vi "6.0.0_Finalization_good_unit.vi"(7 "Data in":T1, 8 "error in (no error)":errorcluster, 9 "AllControls In":T2, 10 "?":T3, 11 "Message Queue out":T4) -> (0 "error out":errorcluster, 1 "Flow":string, 2 "Data":T3, 3 "Message Queue Out":T4, 5 "Data out":T1)   [LabVIEW 2017]
uses:
  Depends/AMC/subVIs/TypeDefs/amc_Message Queue.ctl
  Depends/AMC/subVIs/TypeDefs/amc_Message.ctl
  Depends/Tools/Keyed Array/Tools_KeyedArray KeyedArray.ctl
  Ctrls/Data.ctl
  Ctrls/AllControls.ctl
  Ctrls/CSV_Data.ctl
  DIPC 692 Daemon API/typdef/device_mode.ctl
  Ctrls/PathChoose.ctl
  DIPC 692 Daemon API/typdef/read_nvm_section.ctl
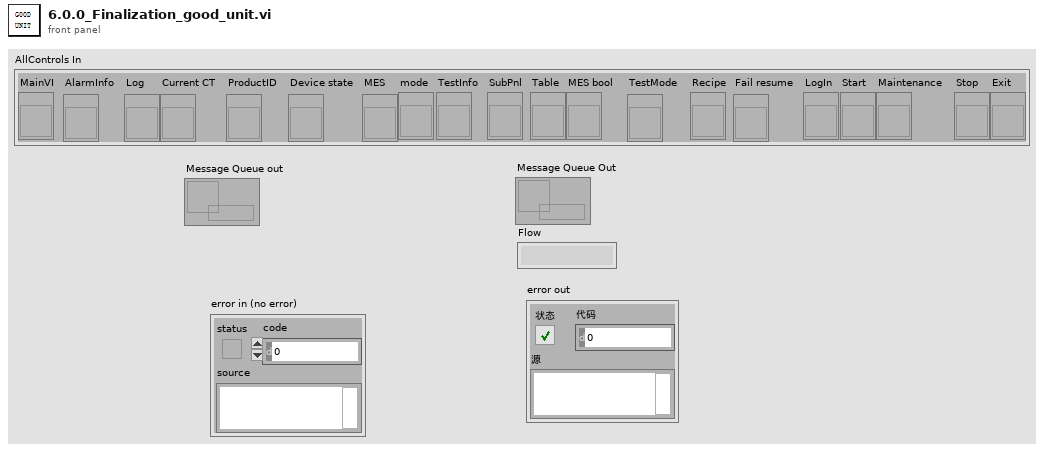
[diagram p1: front panel]
types:
  T1 = typedef "CSV_Data.ctl" = cluster{"Initialisation":cluster{"LMT - Connect UUT (con COM)":string, "LMT - Software Version (rrel)":string, "LMT - Write SKU file (wskuc)":string, "LMT - SKU file name":string, "Connect UUT DDM":string, "Read DDM EOL Timestamp - Mode":string, "Read DDM EOL Timestamp - Timestamp":string, "Read DDM EOL Timestamp - Rig ID":string, "Read DDM EOL Timestamp - Passmark ID":string, "Read DDM EOL Timestamp - Passmark Rev":string, "Software Version before flashing":string, "Read Hardware Serial":string, "UUT DDM SN":string, "Compare DDM SN with MES SN":string, "Backup PCBA Calibration EEPROM Response - CAL":string, "Flash Firmware Version":string, "Check SW Version":string, "Read DDM SW Version after flashing":string, "Set SKU Config":string, "Ready Status":string, "Set Device Mode to EOL":string, "DDM Parameter - Voltage":string, "DDM Parameter - Current":string, "DDM Parameter - Power":string, "DDM Parameter - Speed":string, "DDM Parameter - Pressure":string, "Tester Parameter - Voltage":string, "Tester Parameter - Current":string, "Tester Parameter - Power":string, "Tester Parameter - Ambient Pressure":string, "Tester Parameter - Ambient Temperature":string, "Calculated Parameter - DDM Pressure Corrected":string, "Calculated Parameter - DDM Real Power":string, "Calculated Parameter - Delta V":string}, "BEMF_Calibration":cluster{"Calibration Result - eol_cold_bemf_temp":string, "DDM Ambient Temp":string, "Restriction Plate Diameter":string, "Calibration Result - eol_bemf_mp_cold_coef_a":string, "Calibration Result - eol_bemf_mp_cold_coef_b":string, "Calibration Result - eol_bemf_mp_cold_coef_c":string, "Calibration Result - eol_bemf_lsi_cold_ref_coeffs":string, "Get - Calibration Result - eol_bemf_lsi_speed":string, "Get - Calibration Result - eol_bemf_lsi_integral_0":string, "Calibration Result - eol_bemf_lsi_integral_1":string, "Get - Calibration Result - eol_bemf_lsi_integral_2":string, "Get - Calibration Result - eol_cold_bemf":string, "Get - Calibration Result - eol_cold_bemf_fisf":string, "Finalise Calibration":string, "Compare -Calibration Result - eol_cold_bemf":string, "Compare -Calibration Result - eol_cold_bemf_fisf":string}, "ECO":cluster{"Reset Power Tune":string, "Reset BEMF FISF Calibration":string, "Restriction Plate Diameter":string, "ECO - Stabilisation Time":string, "ECO - DDM Parameter - Voltage":string, "ECO - DDM Parameter - Current":string, "ECO - DDM Parameter - Power":string, "ECO - DDM Parameter - Measured Power":string, "ECO - DDM Parameter - Speed":string, "ECO - DDM Parameter - Pressure":string, "ECO - Tester Parameter - Voltage":string, "ECO - Tester Parameter - Current":string, "ECO - Tester Parameter - Power":string, "ECO - Tester Parameter - Ambient Pressure":string, "ECO - Tester Parameter - Ambient Temperature":string, "ECO - Tester Parameter - Ambient Humidity":string, "ECO - Calculated Parameter - DDM Pressure Corrected":string, "ECO - Calculated Parameter - DDM Real Power":string, "ECO - Calculated Parameter - Delta V":string, "ECO - Calculated Parameter - Flowrate":string, "ECO - Calculated Parameter - Airwatt":string, "ECO - Formula":string, "PT ECO - Power Tune Mode Status":string}, "BOOST":cluster{"Restriction Plate Diameter":string, "BOOST - Stabilisation Time":string, "BOOST - DDM Parameter - Voltage":string, "BOOST - DDM Parameter - Current":string, "BOOST - DDM Parameter - Power":string, "BOOST - DDM Parameter - Measured Power":string, "BOOST - DDM Parameter - Speed":string, "BOOST - DDM Parameter - Pressure":string, "BOOST - Tester Parameter - Voltage":string, "BOOST - Tester Parameter - Current":string, "BOOST - Tester Parameter - Power":string, "BOOST - Tester Parameter - Ambient Pressure":string, "BOOST - Tester Parameter - Ambient Temperature":string, "BOOST - Tester Parameter - Ambient Humidity":string, "BOOST - Calculated Parameter - DDM Pressure Corrected":string, "BOOST - Calculated Parameter - DDM Real Power":string, "BOOST - Calculated Parameter - Delta V":string, "BOOST - Calculated Parameter - Flowrate":string, "BOOST - Calculated Parameter - Airwatt":string, "BOOST - Get AM Presence":string, "Air Muscle Turn Off Status":string, "BOOST - Air Muscle Calculated Parameter - Airwatt B":string, "BOOST - Air Muscle Calculate Airwatt Delta":string, "PT BOOST - Power Tune Mode Status":string, "Finalise Calibration":string, "ECO - Get AW Calibration value":string, "BOOST - Get AW Calibration value":string}, "MAX":cluster{"Restriction Plate Diameter":string, "MAX - Stabilisation Time":string, "Get Average Delta Tmag (LSIdelta_FISFdelta_LSItmag_FISFtmag_IIRtmag)":string, "Get Average Delta Tmag FISF":string, "MAX - DDM Parameter - Voltage":string, "MAX - DDM Parameter - Current":string, "MAX - DDM Parameter - Power":string, "MAX - DDM Parameter - Measured Power":string, "MAX - DDM Parameter - Speed":string, "MAX - DDM Parameter - Pressure":string, "MAX - Tester Parameter - Voltage":string, "MAX - Tester Parameter - Current":string, "MAX - Tester Parameter - Power":string, "MAX - Tester Parameter - Ambient Pressure":string, "MAX - Tester Parameter - Ambient Temperature":string, "MAX - Tester Parameter - Ambient Humidity":string, "MAX - Calculated Parameter - DDM Pressure Corrected":string, "MAX - Calculated Parameter - DDM Real Power":string, "MAX - Calculated Parameter - Delta V":string, "MAX - Calculated Parameter - Flowrate":string, "MAX - Calculated Parameter - Airwatt":string, "MAX_FISF_Check_Average_Delta_Tmag":string, "MAX - FISF - BEMF Finetune Result":string, "MAX tune - Delta P1":string, "MAX tune - Calculated Parameter - Airwatt":string, "Calculate Delta Airwatts - MAX finetune - Delta P2":string, "MAX finetune - DDM Parameter - Voltage":string, "MAX finetune - DDM Parameter - Current":string, "MAX finetune - DDM Parameter - Power":string, "MAX finetune - DDM Parameter - Measured Power":string, "MAX finetune - DDM Parameter - Speed":string, "MAX finetune - DDM Parameter - Pressure":string, "MAX finetune - Tester Parameter - Voltage":string, "MAX finetune - Tester Parameter - Current":string, "MAX finetune - Tester Parameter - Power":string, "MAX finetune - Tester Parameter - Ambient Pressure":string, "MAX finetune - Tester Parameter - Ambient Temperature":string, "MAX finetune - Tester Parameter - Ambient Humidity":string, "MAX finetune - Calculated Parameter - DDM Pressure Corrected":string, "MAX finetune - Calculated Parameter - DDM Real Power":string, "MAX finetune - Calculated Parameter - Delta V":string, "MAX finetune - Calculated Parameter - Flowrate":string, "MAX finetune - Calculated Parameter - Airwatt":string, "Check Derate Result":string, "Delta Tmag FISF":string, "Get Hot BEMF Result":string, "Calculate delta Pressure":string, "Finalise Calibration":string, "Calculate & Check Delta BEMF":string, "Delta P Airwatts Value":string}, "LL":cluster{"DDM Ambient Temp":string, "Restriction Plate Diameter":string, "LL - DDM Parameter - Voltage":string, "LL - DDM Parameter - Current":string, "LL - DDM Parameter - Power":string, "LL - DDM Parameter - Measured Power":string, "LL - DDM Parameter - Speed":string, "LL - DDM Parameter - Pressure":string, "LL - Tester Parameter - Voltage":string, "LL - Tester Parameter - Current":string, "LL - Tester Parameter - Power":string, "LL - DDM Real Power":string, "LL - Calibrate Task Detect LL":string}, "HL":cluster{"HL - DDM Parameter - Voltage":string, "HL - DDM Parameter - Current":string, "HL - DDM Parameter - Power":string, "HL - DDM Parameter - Measured Power":string, "HL - DDM Parameter - Speed":string, "HL - DDM Parameter - Pressure":string, "HL - Tester Parameter - Voltage":string, "HL - Tester Parameter - Current":string, "HL - Tester Parameter - Power":string, "HL - DDM Real Power":string, "HL - Calibrate Task Detect HL":string}, "LH":cluster{"Restriction Plate Diameter":string, "LH - DDM Parameter - Voltage":string, "LH - DDM Parameter - Current":string, "LH - DDM Parameter - Power":string, "LH - DDM Parameter - Measured Power":string, "LH - DDM Parameter - Speed":string, "LH - DDM Parameter - Pressure":string, "LH - Tester Parameter - Voltage":string, "LH - Tester Parameter - Current":string, "LH - Tester Parameter - Power":string, "LH - DDM Real Power":string, "LH - Calibrate Task Detect LH":string}, "HH":cluster{"HH - DDM Parameter - Voltage":string, "HH - DDM Parameter - Current":string, "HH - DDM Parameter - Power":string, "HH - DDM Parameter - Measured Power":string, "HH - DDM Parameter - Speed":string, "HH - DDM Parameter - Pressure":string, "HH - Tester Parameter - Voltage":string, "HH - Tester Parameter - Current":string, "HH - Tester Parameter - Power":string, "HH - DDM Real Power":string, "HH - Calibrate Task Detect HH":string}, "Inlet Blockage Calibration":cluster{"Inlet Blockage Calibration - DDM Parameter - Voltage":string, "Inlet Blockage Calibration - DDM Parameter - Current":string, "Inlet Blockage Calibration - DDM Parameter - Power":string, "Inlet Blockage Calibration - DDM Parameter - Measured Power":string, "Inlet Blockage Calibration - DDM Parameter - Speed":string, "Inlet Blockage Calibration - DDM Parameter - Pressure":string, "Inlet Blockage Calibration - Tester Parameter - Voltage":string, "Inlet Blockage Calibration - Tester Parameter - Current":string, "Inlet Blockage Calibration - Tester Parameter - Power":string, "Inlet Blockage Calibration - DDM Real Power":string, "Calibration Inlet Blockage_E":string, "Finalise Calibration":string, "Get Task Detect LL":string, "Get Task Detect HL":string, "Get Task Detect LH":string, "Get Task Detect HH":string, "Calibration Inlet Blockage":string, "Calibration eol cold bemf temp":string}, "GOOD":cluster{"GOOD UNIT - Clear EEPROM Error Log":string, "GOOD UNIT - Write Product Timestamp - Mode":string, "GOOD UNIT - Write Product Timestamp - Timestamp":string, "GOOD UNIT - Write Product Timestamp - Rig ID":string, "GOOD UNIT - Write Product Timestamp - Passmark ID":string, "GOOD UNIT - Write Product Timestamp - Passmark Rev":string, "GOOD UNIT - Set Device Mode to PROD":string, "GOOD UNIT - Backup PCBA Calibration EEPROM Response":string, "GOOD UNIT - Check Security Bit":string, "GOOD UNIT - Set Calibration Lock":string, "GOOD UNIT - Get_Calibration_Lock":string, "GOOD UNIT - Disconnect UUT":string}, "NG":cluster{"NG UNIT - Read NVM Error":string, "NG UNIT - Set Device Mode to FCT":string, "NG UNIT - Backup PCBA Calibration EEPROM Response - CAL":string, "NG UNIT - Backup PCBA Calibration EEPROM Response - ERROR":string, "NG UNIT - Backup PCBA Calibration EEPROM Response - USAGE":string, "NG UNIT - Disconnect UUT":string}, "SN":string, "Table":string[][], "Count":cluster{"Total":i32, "OK":i32, "NG":i32, "Yield":dbl}, "Start Time":timestamp, "daemon reference":refnum<k5>, "CT":dbl, "Config":string[][], "OK/NG":bool, "Station ID":string, "MES DDM SN":string, "MES PCBA SN":string, "Retest":string, "UID":string, "Initialisation_Status":cluster{"LMT - Connect UUT (con COM)":string, "LMT - Software Version (rrel)":string, "LMT - Write SKU file (wskuc)":string, "LMT - SKU file name":string, "Connect UUT DDM":string, "Read DDM EOL Timestamp - Mode":string, "Read DDM EOL Timestamp - Timestamp":string, "Read DDM EOL Timestamp - Rig ID":string, "Read DDM EOL Timestamp - Passmark ID":string, "Read DDM EOL Timestamp - Passmark Rev":string, "Software Version before flashing":string, "Read Hardware Serial":string, "UUT DDM SN":string, "Compare DDM SN with MES SN":string, "Backup PCBA Calibration EEPROM Response - CAL":string, "Flash Firmware Version":string, "Check SW Version":string, "Read DDM SW Version after flashing":string, "Set SKU Config":string, "Ready Status":string, "Set Device Mode to EOL":string, "DDM Parameter - Voltage":string, "DDM Parameter - Current":string, "DDM Parameter - Power":string, "DDM Parameter - Speed":string, "DDM Parameter - Pressure":string, "Tester Parameter - Voltage":string, "Tester Parameter - Current":string, "Tester Parameter - Power":string, "Tester Parameter - Ambient Pressure":string, "Tester Parameter - Ambient Temperature":string, "Calculated Parameter - DDM Pressure Corrected":string, "Calculated Parameter - DDM Real Power":string, "Calculated Parameter - Delta V":string}, "BEMF_Calibration_Status":cluster{"Calibration Result - eol_cold_bemf_temp":string, "DDM Ambient Temp":string, "Restriction Plate Diameter":string, "Calibration Result - eol_bemf_mp_cold_coef_a":string, "Calibration Result - eol_bemf_mp_cold_coef_b":string, "Calibration Result - eol_bemf_mp_cold_coef_c":string, "Calibration Result - eol_bemf_lsi_cold_ref_coeffs":string, "Get - Calibration Result - eol_bemf_lsi_speed":string, "Get - Calibration Result - eol_bemf_lsi_integral_0":string, "Calibration Result - eol_bemf_lsi_integral_1":string, "Get - Calibration Result - eol_bemf_lsi_integral_2":string, "Get - Calibration Result - eol_cold_bemf":string, "Get - Calibration Result - eol_cold_bemf_fisf":string, "Finalise Calibration":string, "Compare -Calibration Result - eol_cold_bemf":string, "Compare -Calibration Result - eol_cold_bemf_fisf":string}, "ECO_Status":cluster{"Reset Power Tune":string, "Reset BEMF FISF Calibration":string, "Restriction Plate Diameter":string, "ECO - Stabilisation Time":string, "ECO - DDM Parameter - Voltage":string, "ECO - DDM Parameter - Current":string, "ECO - DDM Parameter - Power":string, "ECO - DDM Parameter - Measured Power":string, "ECO - DDM Parameter - Speed":string, "ECO - DDM Parameter - Pressure":string, "ECO - Tester Parameter - Voltage":string, "ECO - Tester Parameter - Current":string, "ECO - Tester Parameter - Power":string, "ECO - Tester Parameter - Ambient Pressure":string, "ECO - Tester Parameter - Ambient Temperature":string, "ECO - Tester Parameter - Ambient Humidity":string, "ECO - Calculated Parameter - DDM Pressure Corrected":string, "ECO - Calculated Parameter - DDM Real Power":string, "ECO - Calculated Parameter - Delta V":string, "ECO - Calculated Parameter - Flowrate":string, "ECO - Calculated Parameter - Airwatt":string, "ECO - Formula":string, "PT ECO - Power Tune Mode Status":string}, "BOOST_Status":cluster{"Restriction Plate Diameter":string, "BOOST - Stabilisation Time":string, "BOOST - DDM Parameter - Voltage":string, "BOOST - DDM Parameter - Current":string, "BOOST - DDM Parameter - Power":string, "BOOST - DDM Parameter - Measured Power":string, "BOOST - DDM Parameter - Speed":string, "BOOST - DDM Parameter - Pressure":string, "BOOST - Tester Parameter - Voltage":string, "BOOST - Tester Parameter - Current":string, "BOOST - Tester Parameter - Power":string, "BOOST - Tester Parameter - Ambient Pressure":string, "BOOST - Tester Parameter - Ambient Temperature":string, "BOOST - Tester Parameter - Ambient Humidity":string, "BOOST - Calculated Parameter - DDM Pressure Corrected":string, "BOOST - Calculated Parameter - DDM Real Power":string, "BOOST - Calculated Parameter - Delta V":string, "BOOST - Calculated Parameter - Flowrate":string, "BOOST - Calculated Parameter - Airwatt":string, "BOOST - Get AM Presence":string, "Air Muscle Turn Off Status":string, "BOOST - Air Muscle Calculated Parameter - Airwatt B":string, "BOOST - Air Muscle Calculate Airwatt Delta":string, "PT BOOST - Power Tune Mode Status":string, "Finalise Calibration":string, "ECO - Get AW Calibration value":string, "BOOST - Get AW Calibration value":string}, "MAX_Status":cluster{"Restriction Plate Diameter":string, "MAX - Stabilisation Time":string, "Get Average Delta Tmag (LSIdelta_FISFdelta_LSItmag_FISFtmag_IIRtmag)":string, "Get Average Delta Tmag FISF":string, "MAX - DDM Parameter - Voltage":string, "MAX - DDM Parameter - Current":string, "MAX - DDM Parameter - Power":string, "MAX - DDM Parameter - Measured Power":string, "MAX - DDM Parameter - Speed":string, "MAX - DDM Parameter - Pressure":string, "MAX - Tester Parameter - Voltage":string, "MAX - Tester Parameter - Current":string, "MAX - Tester Parameter - Power":string, "MAX - Tester Parameter - Ambient Pressure":string, "MAX - Tester Parameter - Ambient Temperature":string, "MAX - Tester Parameter - Ambient Humidity":string, "MAX - Calculated Parameter - DDM Pressure Corrected":string, "MAX - Calculated Parameter - DDM Real Power":string, "MAX - Calculated Parameter - Delta V":string, "MAX - Calculated Parameter - Flowrate":string, "MAX - Calculated Parameter - Airwatt":string, "MAX_FISF_Check_Average_Delta_Tmag":string, "MAX - FISF - BEMF Finetune Result":string, "MAX tune - Delta P1":string, "MAX tune - Calculated Parameter - Airwatt":string, "Calculate Delta Airwatts - MAX finetune - Delta P2":string, "MAX finetune - DDM Parameter - Voltage":string, "MAX finetune - DDM Parameter - Current":string, "MAX finetune - DDM Parameter - Power":string, "MAX finetune - DDM Parameter - Measured Power":string, "MAX finetune - DDM Parameter - Speed":string, "MAX finetune - DDM Parameter - Pressure":string, "MAX finetune - Tester Parameter - Voltage":string, "MAX finetune - Tester Parameter - Current":string, "MAX finetune - Tester Parameter - Power":string, "MAX finetune - Tester Parameter - Ambient Pressure":string, "MAX finetune - Tester Parameter - Ambient Temperature":string, "MAX finetune - Tester Parameter - Ambient Humidity":string, "MAX finetune - Calculated Parameter - DDM Pressure Corrected":string, "MAX finetune - Calculated Parameter - DDM Real Power":string, "MAX finetune - Calculated Parameter - Delta V":string, "MAX finetune - Calculated Parameter - Flowrate":string, "MAX finetune - Calculated Parameter - Airwatt":string, "Check Derate Result":string, "Delta Tmag FISF":string, "Get Hot BEMF Result":string, "Calculate delta Pressure":string, "Finalise Calibration":string, "Calculate & Check Delta BEMF":string, "Delta P Airwatts Value":string}, "LL_Status":cluster{"DDM Ambient Temp":string, "Restriction Plate Diameter":string, "LL - DDM Parameter - Voltage":string, "LL - DDM Parameter - Current":string, "LL - DDM Parameter - Power":string, "LL - DDM Parameter - Measured Power":string, "LL - DDM Parameter - Speed":string, "LL - DDM Parameter - Pressure":string, "LL - Tester Parameter - Voltage":string, "LL - Tester Parameter - Current":string, "LL - Tester Parameter - Power":string, "LL - DDM Real Power":string, "LL - Calibrate Task Detect LL":string}, "HL_Status":cluster{"HL - DDM Parameter - Voltage":string, "HL - DDM Parameter - Current":string, "HL - DDM Parameter - Power":string, "HL - DDM Parameter - Measured Power":string, "HL - DDM Parameter - Speed":string, "HL - DDM Parameter - Pressure":string, "HL - Tester Parameter - Voltage":string, "HL - Tester Parameter - Current":string, "HL - Tester Parameter - Power":string, "HL - DDM Real Power":string, "HL - Calibrate Task Detect HL":string}, "LH_Status":cluster{"Restriction Plate Diameter":string, "LH - DDM Parameter - Voltage":string, "LH - DDM Parameter - Current":string, "LH - DDM Parameter - Power":string, "LH - DDM Parameter - Measured Power":string, "LH - DDM Parameter - Speed":string, "LH - DDM Parameter - Pressure":string, "LH - Tester Parameter - Voltage":string, "LH - Tester Parameter - Current":string, "LH - Tester Parameter - Power":string, "LH - DDM Real Power":string, "LH - Calibrate Task Detect LH":string}, "HH_Status":cluster{"HH - DDM Parameter - Voltage":string, "HH - DDM Parameter - Current":string, "HH - DDM Parameter - Power":string, "HH - DDM Parameter - Measured Power":string, "HH - DDM Parameter - Speed":string, "HH - DDM Parameter - Pressure":string, "HH - Tester Parameter - Voltage":string, "HH - Tester Parameter - Current":string, "HH - Tester Parameter - Power":string, "HH - DDM Real Power":string, "HH - Calibrate Task Detect HH":string}, "Inlet Blockage Calibration_Status":cluster{"Inlet Blockage Calibration - DDM Parameter - Voltage":string, "Inlet Blockage Calibration - DDM Parameter - Current":string, "Inlet Blockage Calibration - DDM Parameter - Power":string, "Inlet Blockage Calibration - DDM Parameter - Measured Power":string, "Inlet Blockage Calibration - DDM Parameter - Speed":string, "Inlet Blockage Calibration - DDM Parameter - Pressure":string, "Inlet Blockage Calibration - Tester Parameter - Voltage":string, "Inlet Blockage Calibration - Tester Parameter - Current":string, "Inlet Blockage Calibration - Tester Parameter - Power":string, "Inlet Blockage Calibration - DDM Real Power":string, "Calibration Inlet Blockage_E":string, "Finalise Calibration":string, "Get Task Detect LL":string, "Get Task Detect HL":string, "Get Task Detect LH":string, "Get Task Detect HH":string, "Calibration Inlet Blockage":string, "Calibration eol cold bemf temp":string}, "GOOD_Status":cluster{"GOOD UNIT - Clear EEPROM Error Log":string, "GOOD UNIT - Write Product Timestamp - Mode":string, "GOOD UNIT - Write Product Timestamp - Timestamp":string, "GOOD UNIT - Write Product Timestamp - Rig ID":string, "GOOD UNIT - Write Product Timestamp - Passmark ID":string, "GOOD UNIT - Write Product Timestamp - Passmark Rev":string, "GOOD UNIT - Set Device Mode to PROD":string, "GOOD UNIT - Backup PCBA Calibration EEPROM Response":string, "GOOD UNIT - Check Security Bit":string, "GOOD UNIT - Set Calibration Lock":string, "GOOD UNIT - Get_Calibration_Lock":string, "GOOD UNIT - Disconnect UUT":string}, "NG_Status":cluster{"NG UNIT - Read NVM Error":string, "NG UNIT - Set Device Mode to FCT":string, "NG UNIT - Backup PCBA Calibration EEPROM Response - CAL":string, "NG UNIT - Backup PCBA Calibration EEPROM Response - ERROR":string, "NG UNIT - Backup PCBA Calibration EEPROM Response - USAGE":string, "NG UNIT - Disconnect UUT":string}, "SKU":string, "Plate_Diameter":string, "Alarm":string}
  T2 = typedef "AllControls.ctl" = cluster{"MainVI":refnum<vi>, "AlarmInfo":refnum<vi>, "Log":refnum<vi>, "Current CT":refnum<vi>, "ProductID":refnum<vi>, "Device state":refnum<vi>, "MES":refnum<vi>, "mode":refnum<vi>, "TestInfo":refnum<vi>, "SubPnl":refnum<vi>, "Table":refnum<vi>, "MES bool":refnum<vi>, "TestMode":refnum<vi>, "Recipe":refnum<vi>, "Fail resume":refnum<vi>, "LogIn":refnum<vi>, "Start":refnum<vi>, "Maintenance":refnum<vi>, "Stop":refnum<vi>, "Exit":refnum<vi>}
  T3 = typedef "Data.ctl" = cluster{"Initialisation":cluster{"DDM_Parameter":dbl[], "DDM_Parameter_status":bool[], "Get_Tester_Parameter":dbl[], "Get_Tester_Parameter_status":bool[], "Cal_Tester_Parameter":dbl[], "Cal_Tester_Parameter_status":bool[], "sw_version_before_status":bool, "sw_version_after_status":bool, "Set_SKU_Config_With_LMT_status":bool, "FCT_timestamp_status":bool, "LMT_Connect_to_UUT_status":bool}, "BEMF_Calibration":cluster{"Read_ambient_temperature":dbl, "Calibration_Vaule":dbl[], "Calibration_Vaule _B":dbl[], "Calibration_Vaule_status":bool[], "Calibration_Vaule_B_status":bool[]}, "ECO":cluster{"DDM_Parameter":dbl[], "DDM_Parameter_status":bool[], "Get_Tester_Parameter":dbl[], "Get_Tester_Parameter_status":bool[], "Cal_Tester_Parameter":dbl[], "Cal_Tester_Parameter_status":bool[], "DDM_Parameter_after_power_tune":dbl[], "Get_Tester_Parameter_after_power_tune":dbl[], "Cal_Tester_Parameter_after_power_tune":dbl[], "Cal_Tester_Parameter_after_power_tune_status":bool[], "Delta_P":dbl}, "BOOST":cluster{"DDM_Parameter":dbl[], "DDM_Parameter_status":bool[], "Get_Tester_Parameter":dbl[], "Get_Tester_Parameter_status":bool[], "Cal_Tester_Parameter":dbl[], "Cal_Tester_Parameter_status":bool[], "DDM_Parameter_after_power_tune":dbl[], "Get_Tester_Parameter_after_power_tune":dbl[], "Cal_Tester_Parameter_after_power_tune":dbl[], "Cal_Tester_Parameter_after_power_tune_status":bool[], "airwatts_am_off":dbl, "AW_Delta_(AM_on_and_off)":dbl, "AW_Delta_(AM_on_and_off)_Status":bool, "Delta_P":dbl}, "MAX":cluster{"Average_Tmag_Data":cluster{"LSI Delta in degC":dbl, "FISF Delta in degc":dbl, "LSI Tmag in degC":dbl, "Fisf Tmag in degC":dbl, "IIR Tmag in degC":dbl}, "DDM_Parameter":dbl[], "DDM_Parameter_status":bool[], "Get_Tester_Parameter":dbl[], "Get_Tester_Parameter_status":bool[], "Cal_Tester_Parameter":dbl[], "BEMF_Finetune":cluster{"eol_bemf_mp_cold_coef_c":dbl, "eol_cold_bemf_fisf_offset":dbl}, "AW_Tune":cluster{"delta_P1":dbl, "delta_P_Setting":dbl}, "DDM_Parameter_after_Airwatts_Tune":dbl[], "Get_Tester_Parameter_after_Airwatts_Tune":dbl[], "Cal_Tester_Parameter_after_Airwatts_Tune":dbl[], "DDM_Parameter_after_Airwatts_Finetune":dbl[], "Get_Tester_Parameter_after_Airwatts_Finetune":dbl[], "Cal_Tester_Parameter_after_Airwatts_Finetune":dbl[], "AW_Finetune":cluster{"delta_P2":dbl, "delta_P_Setting":dbl}, "Delta_Tmag_after_tune":cluster{"LSI Delta in degC":dbl, "FISF Delta in degc":dbl, "LSI Tmag in degC":dbl, "Fisf Tmag in degC":dbl, "IIR Tmag in degC":dbl}, "Hot Bemf in mV":dbl, "DDM_Pressure":dbl, "Delta_Pressure":dbl, " Cold Bemf in mV":dbl, " delta Bemf":dbl, " delta p":dbl, "Delta_Pressure_status":bool, " delta Bemf_status":bool, "LSI Delta in degC_status":bool, "FISF Delta in degc_status":bool, "Max_check_derate_status_status":bool, "Average_All_data":dbl[][], "Average_Tmag_Data_status":bool[], "Average_Tmag_Data_after_tune_status":bool[], "Cal_Tester_Parameter_status":bool[], "Cal_Tester_Parameter_status_after_Airwatts_Tune":bool[], "Cal_Tester_Parameter_status_after_Airwatts_FineTune":bool[]}, "Task_Detect_Calib":cluster{"LL":cluster{"DDM_Parameter":dbl[], "DDM_Parameter_status":bool[], "Get_Tester_Parameter":dbl[], "Get_Tester_Parameter_status":bool[], "Set_task_detect_A":dbl, "Set_task_detect_A_Status":bool}, "HL":cluster{"DDM_Parameter":dbl[], "DDM_Parameter_status":bool[], "Get_Tester_Parameter":dbl[], "Get_Tester_Parameter_status":bool[], "Set_task_detect_B":dbl, "Set_task_detect_B_Status":bool}, "LH":cluster{"DDM_Parameter":dbl[], "DDM_Parameter_status":bool[], "Get_Tester_Parameter":dbl[], "Get_Tester_Parameter_status":bool[], "Set_task_detect_C":dbl, "Set_task_detect_C_Status":bool}, "HH":cluster{"DDM_Parameter":dbl[], "DDM_Parameter_status":bool[], "Get_Tester_Parameter":dbl[], "Get_Tester_Parameter_status":bool[], "Set_task_detect_D":dbl, "Read_and_check_calibration_Status":bool[], "Set_task_detect_D_Status":bool}, "Get_eol_inlet_blockage_E":dbl, "Calib_vaule":cluster{"Get_task_detect_LL":dbl, "Get_task_detect_HL":dbl, "Get_task_detect_LH":dbl, "Get_task_detect_HH":dbl, "eol_inlet_blockage":dbl, "eol_code_bemf_temp":dbl}, "calibrated temp":dbl, "Inlet_Blockage_Calibration":cluster{"DDM_Parameter":dbl[], "DDM_Parameter_status":bool[], "Get_Tester_Parameter":dbl[], "Get_Tester_Parameter_status":bool[]}, "Get_eol_inlet_blockage_E_Status":bool}, "good":cluster{"Write_Product_TS":cluster{"TIMESTAMP":i64, "RIG_ID":i64, "PASSMARK_ID":i64, "PASSMARK_REV":i64}, "Read_Product_TS":cluster{"TIMESTAMP":i64, "RIG_ID":i64, "PASSMARK_ID":i64, "PASSMARK_REV":i64}, "Good_Check_Secuity_Bit_Stauts":bool}}
  T4 = typedef "amc_Message Queue.ctl" = refnum<queue>
  T5 = typedef "TesterInfo.ctl" = cluster{"Station Name":string, "Station Code":string, "ES NO.":string, "Tester ID":string, "PassMark Revision":string, "Rig ID":string, "Deamon_vision":string, "Project Name":string, "FFTesterPath":path, "Enable_User":bool, "Mode":enum16{"682"}, "MES":bool}
  T6 = typedef "HD Config.ctl" = cluster{" PC":cluster{"PC Address":u8[], "PC Port":i32}, "FCO":cluster{"COM":refnum<visa-resource-name>, "Baudrate":u32}, "DC Power ":cluster{"COM":refnum<visa-resource-name>, "Baudrate":u32}, "PW3336":cluster{"COM":refnum<visa-resource-name>, "Baudrate":u32}, "Lefoo":cluster{"COM":refnum<visa-resource-name>, "Baudrate":u32}, "AI Model":cluster{"COM":refnum<visa-resource-name>, "Baudrate":u32}, "DIPC":cluster{"COM":refnum<visa-resource-name>}, "RFID":cluster{"IP Address":string, "Port":u16, "Retry":u16}, "Motor":cluster{"COM":refnum<visa-resource-name>, "Baudrate":u32}, "Fail_resume_mode":bool, "GRR":bool}
  T7 = cluster{"TIMESTAMP":string, "RIG_ID":string, "PASSMARK_ID":string, "PASSMARK_REV":string}
  T8 = cluster{"TIMESTAMP":i64, "RIG_ID":i64, "PASSMARK_ID":i64, "PASSMARK_REV":i64}
  T9 = typedef "device_mode.ctl" = enum16{"FCT", "EOL", "PROD"}
  T10 = typedef "PathChoose.ctl" = enum16{"OperatorLog", "AutoRunLog", "AlmLog", "TestData", "AllTestData", "backup_nvm", "backup_before_flashing"}
  T11 = enum16{"open", "replace", "create", "open or create", "replace or create", "replace or create with confirmation"}
  T12 = typedef "read_nvm_section.ctl" = enum16{"CAL", "ERROR", "USAGE"}
  T13 = cluster{"[0]":i64, "[1]":i64, "[2]":i64, "[3]":i64}
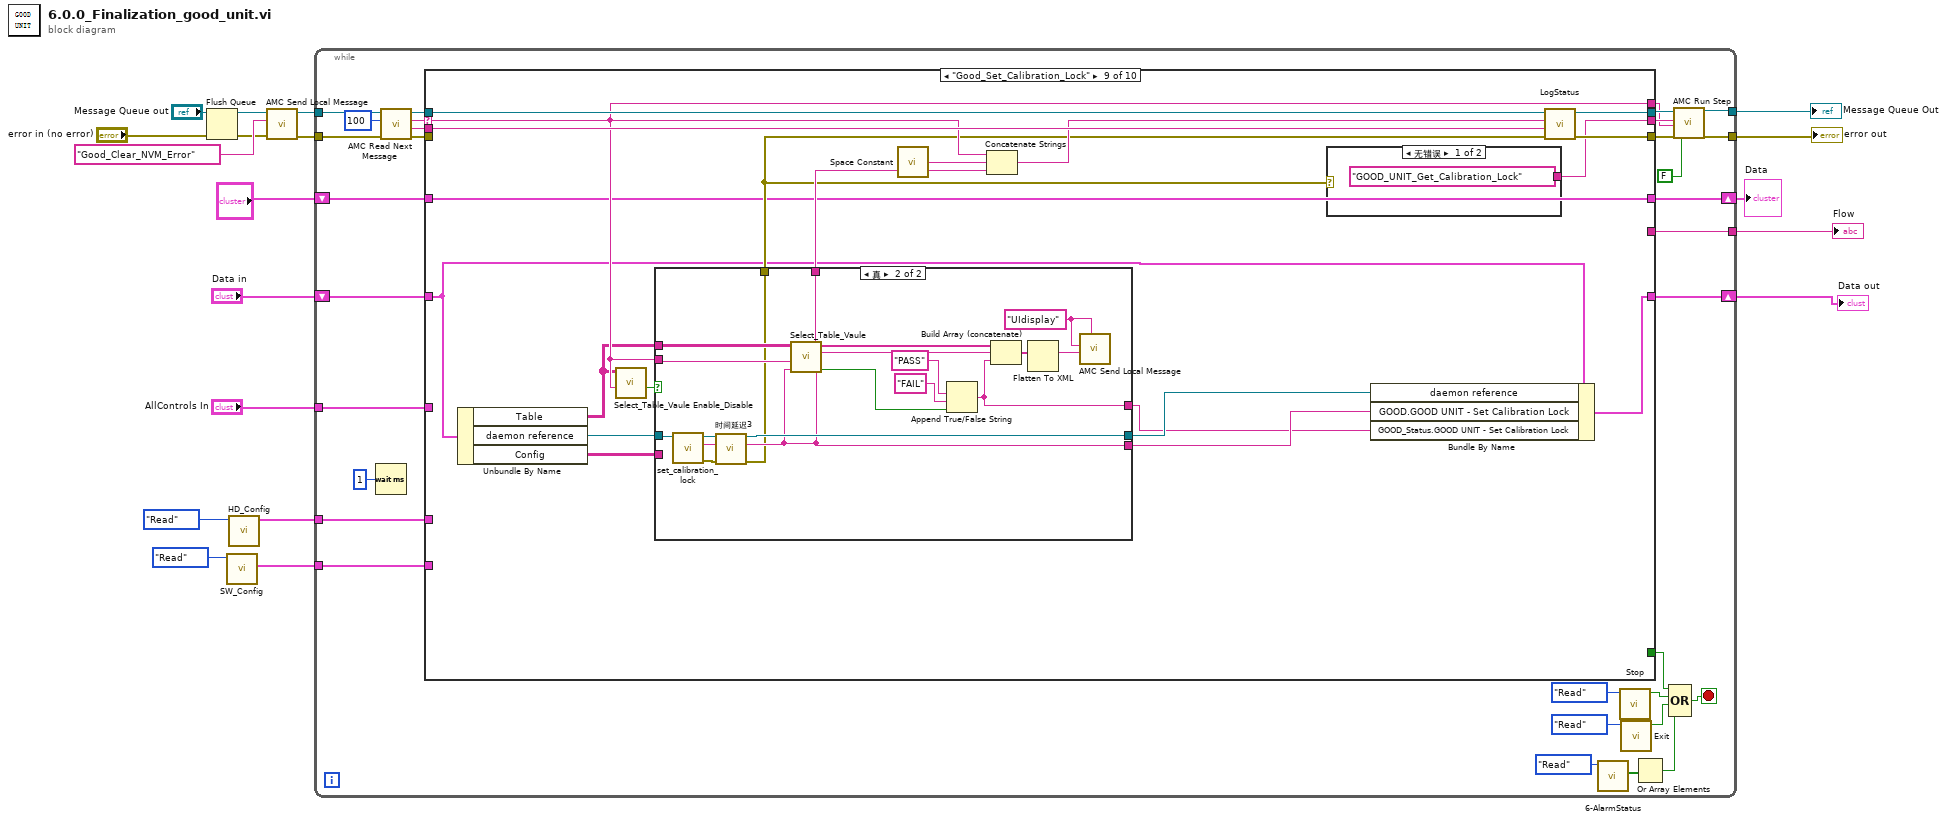
[diagram p0: block diagram]
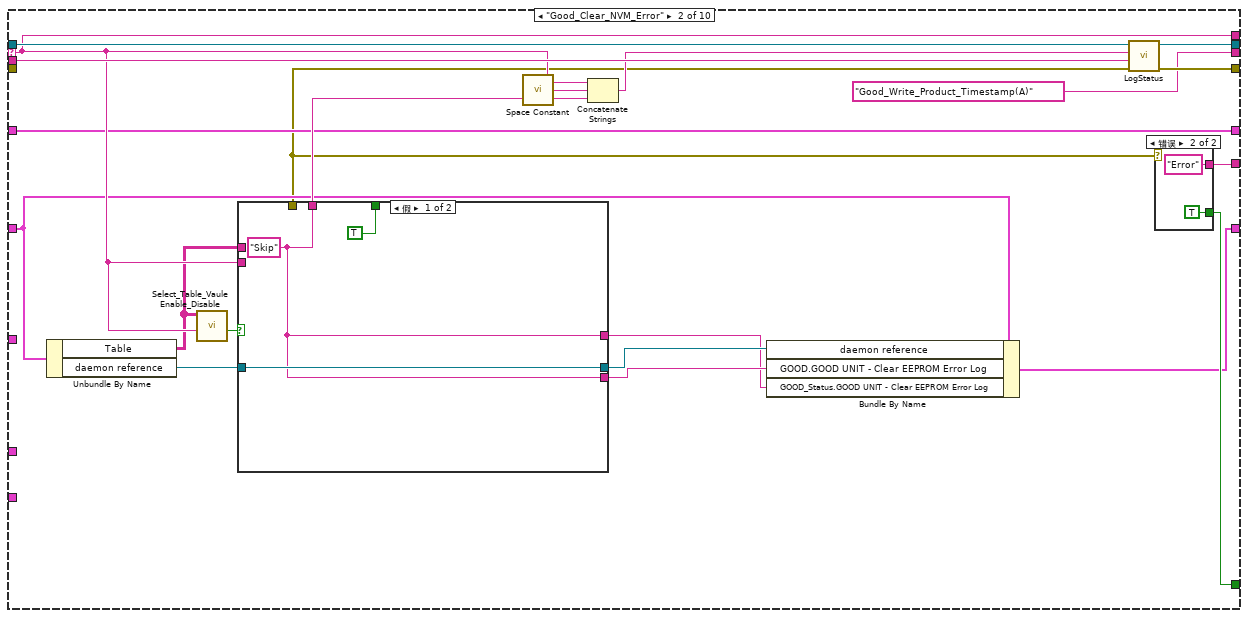
[diagram p3: hidden frame]
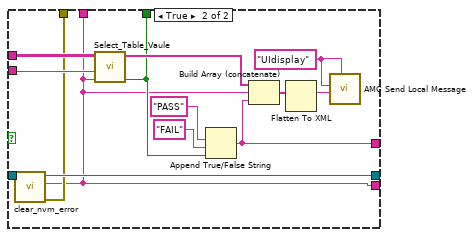
[diagram p5: hidden frame]
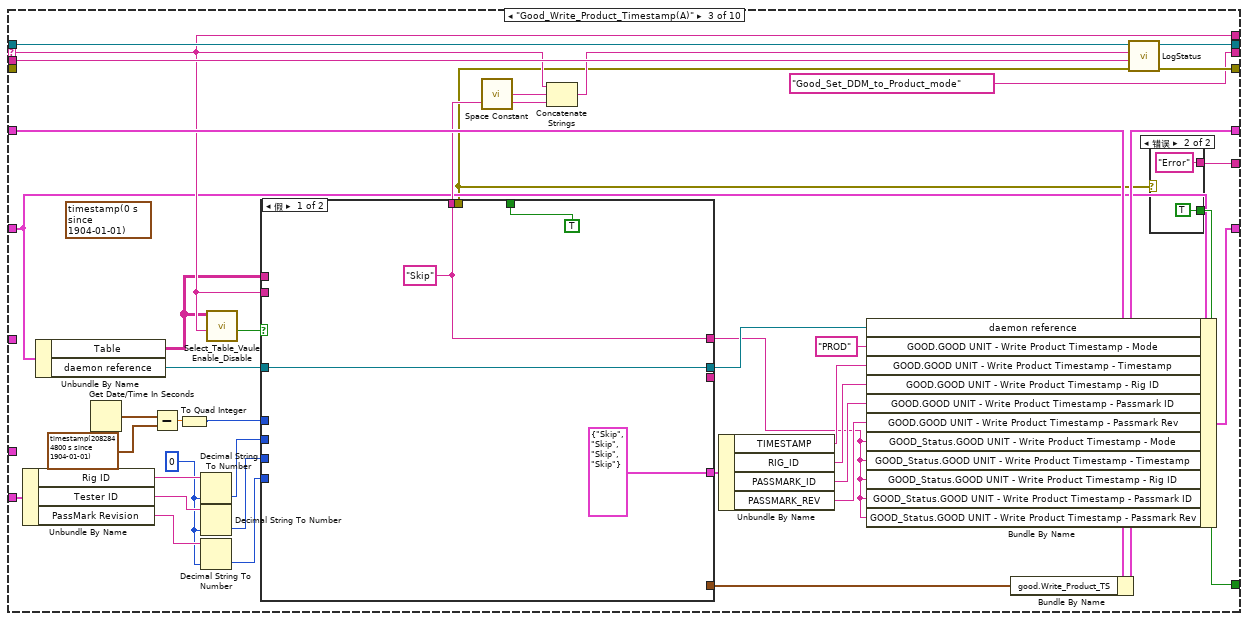
[diagram p6: hidden frame]
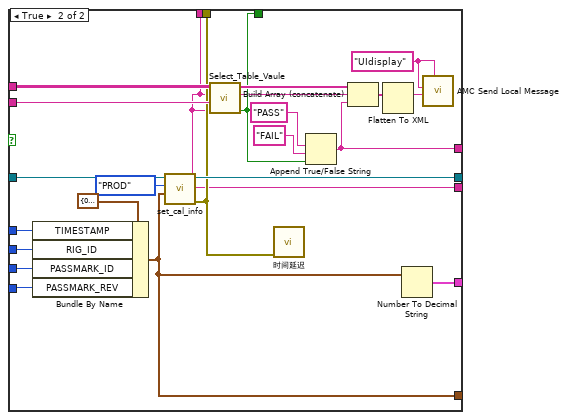
[diagram p8: hidden frame]
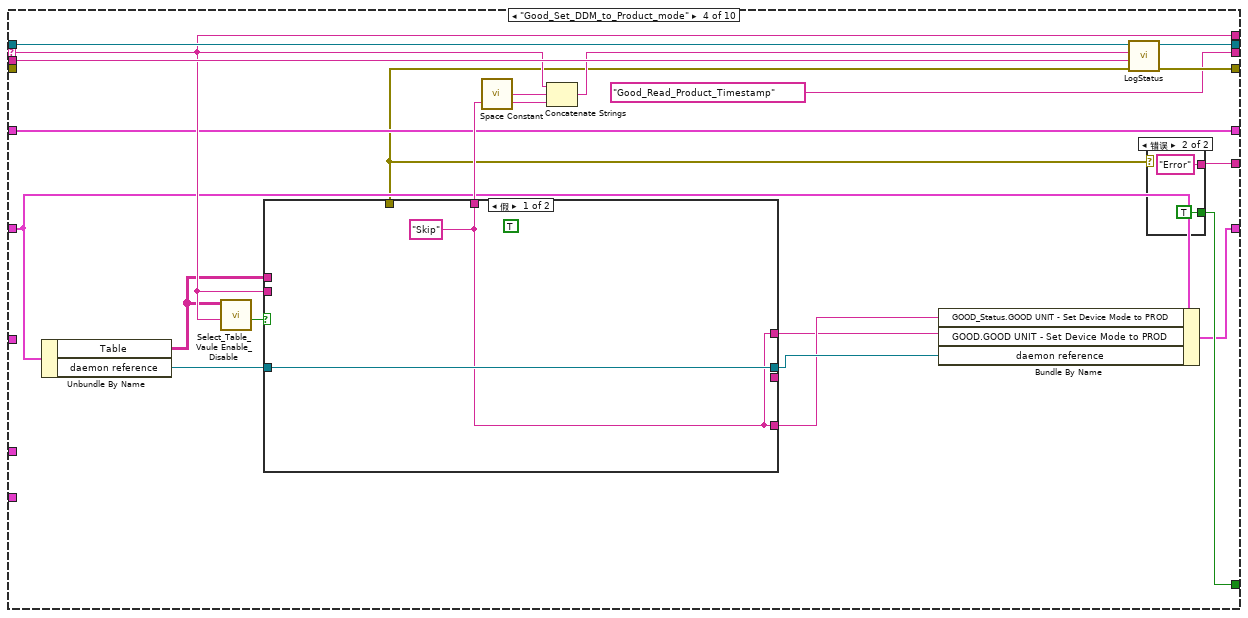
[diagram p9: hidden frame]
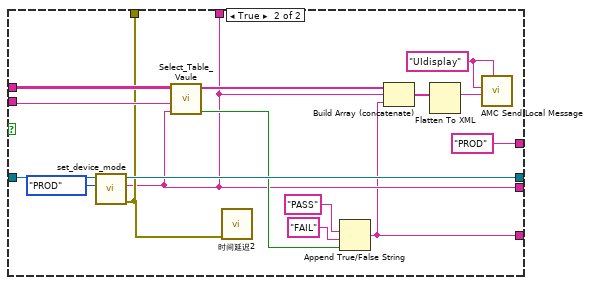
[diagram p11: hidden frame]
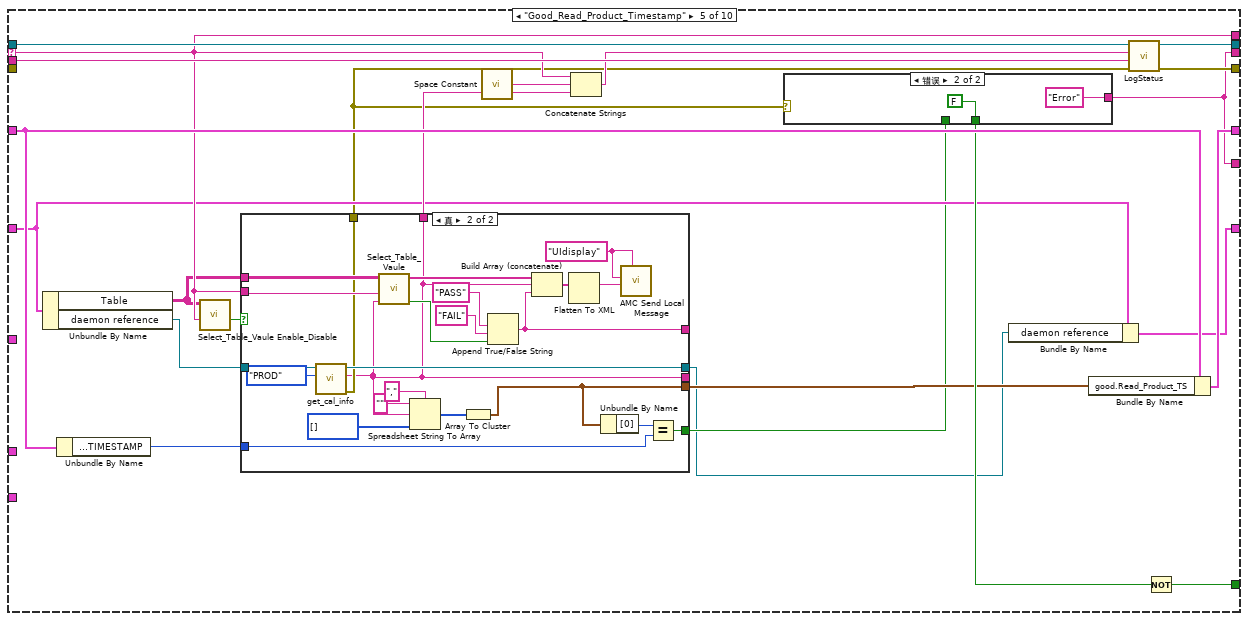
[diagram p12: hidden frame]
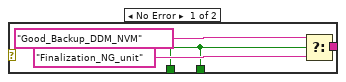
[diagram p13: hidden frame]
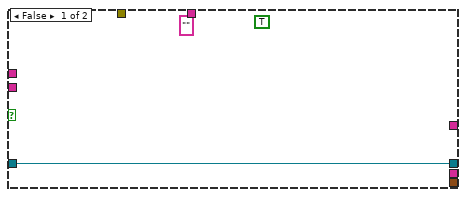
[diagram p14: hidden frame]
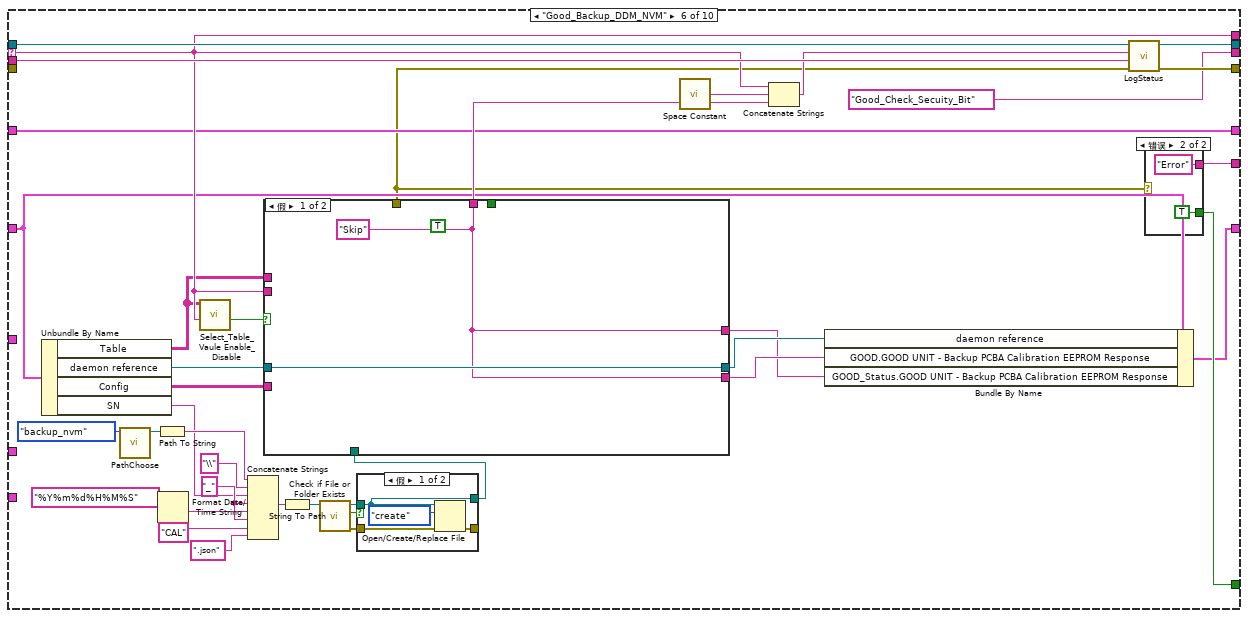
[diagram p15: hidden frame]
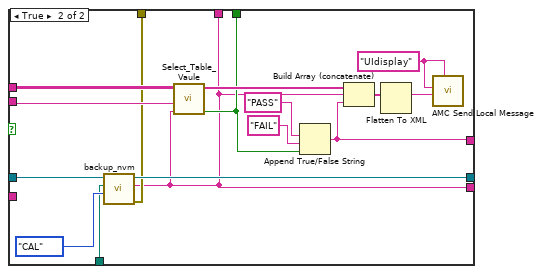
[diagram p18: hidden frame]
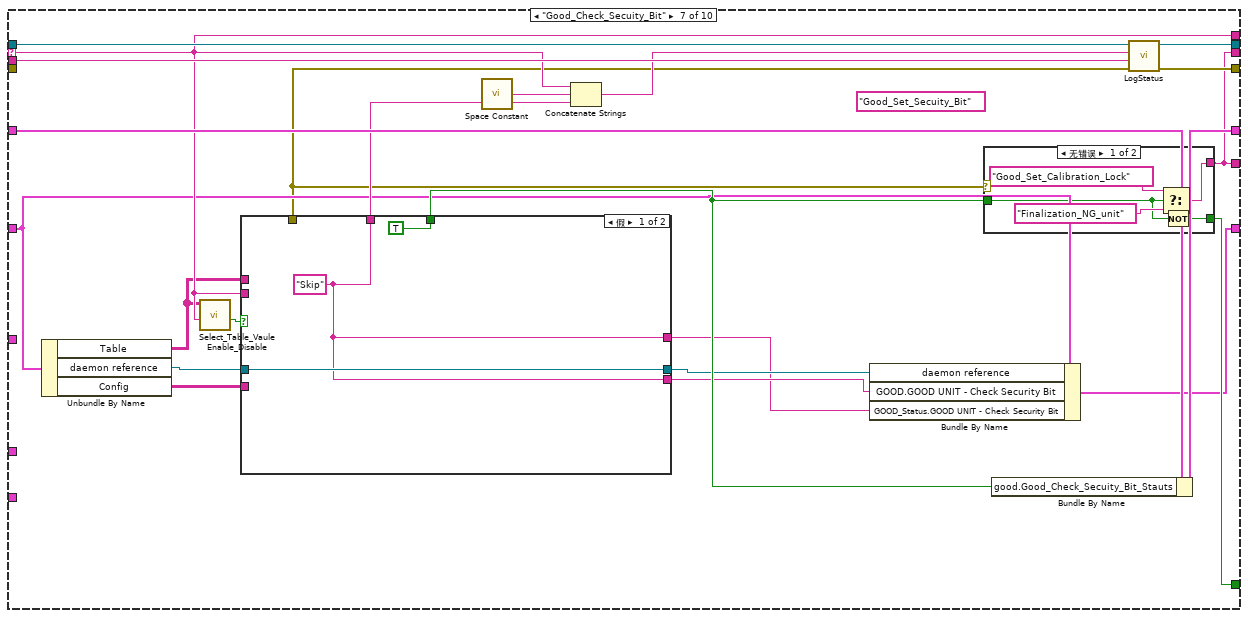
[diagram p19: hidden frame]
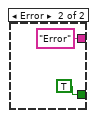
[diagram p20: hidden frame]
diagram:
  n1 = Flush Queue(queue="Message Queue out") -> (queue out=w4:T4)  [unwired: 1 in, 2 out]
  n2 = call "SW_Config.vi"("Step"=enum16{"Initial", "Write", "Read"}."Read") -> ("SW Config out"=w7:T5)  [unwired: 9 in, 1 out]
  n3 = call "HD_Config.vi"("Step"=enum16{"Initial", "Write", "Read"}."Read") -> ("HD Config out"=w10:T6)  [unwired: 9 in, 1 out]
  n4 = call "AMC Send Local Message.vi"("error in (no error)"="error in (no error)", "Message Name"="Good_Clear_NVM_Error", "Message Queue in"=w4) -> ("error out"=w15:errorcluster, "Message Queue out"=w16:T4)  [unwired: 7 in]
  n5 = while {
    tunnel: w16 -> [w50]
    tunnel: [w46] -> w6
    tunnel: w15 -> [w44]
    tunnel: [w41] -> w5
    shift-right: [w37] -> w12
    shift-left: "?" -> [w38]
    tunnel: w10 -> [w36]
    tunnel: [w32] -> w9
    tunnel: w7 -> [w31]
    shift-right: [w22] -> w1
    shift-left: "Data in" -> [w24]
    tunnel: "AllControls In" -> [w23]
    stop <- w25 stop-if-true
    n6 = Wait (ms)(milliseconds to wait=u32 1 ("等待时间（毫秒）")) -> ()  [unwired: 1 out]
    n7 = call "AMC Read Next Message.vi"("error in (no error)"=w44, "timeout (1ms)"=100, "Message Queue in"=w50) -> ("error out"=w43:errorcluster, "Message Value"=w34:string, "Message Name"=w48:string, "Message Queue out"=w49:T4)  [unwired: 1 in, 4 out]
    n8 = case shown="\"Good_Set_Calibration_Lock\"" w48 {
      selector: w48 -> [_ w67 w123 w173 w215 w284 w330 w375 w422 w468]
      tunnel: w49 -> [w54 w74 w132 w180 w222 w290 w338 w381 w428 w474]
      tunnel: [w54 w74 w132 w180 w222 w290 w338 w381 w428 w474] -> w47
      tunnel: w43 -> [w53 _ _ _ _ _ _ _ _ _]
      tunnel: [w53 w73 w131 w179 w221 w289 w337 w380 w427 w473] -> w42
      tunnel: [_ w63 w111 w169 w212 w277 w327 w370 _ TRUE] -> w26
      tunnel: w38 -> [w52 w61 w128 w167 w219 w260 w334 w368 w412 w456]
      tunnel: [w52 w61 w127 w167 w218 w260 w333 w368 w412 w456] -> w37
      tunnel: w34 -> [_ w72 w130 w178 w220 w288 w336 w379 w426 w472]
      tunnel: [_ w67 w123 w173 w215 w284 w330 w375 w422 w468] -> w33
      tunnel: w36 -> [_ _ _ _ _ _ _ _ _ _]
      tunnel: [_ "Good_Write_Product_Timestamp(A)" "Good_Set_DDM_to_Product_mode" "Good_Read_Product_Timestamp" w213 "Good_Check_Secuity_Bit" w323 "Good_Set_Calibration_Lock" w419 w463] -> w35
      tunnel: [_ w64 w112 w170 w213 w278 w323 w371 _ w463] -> w32
      tunnel: w31 -> [_ _ w120 _ _ _ _ _ _ _]
      tunnel: w24 -> [w51 w60 w104 w166 w206 w259 w322 w367 w415 w462]
      tunnel: w23 -> [_ _ _ _ _ _ _ _ _ _]
      tunnel: [w51 w59 w100 w164 w201 w256 w319 w364 w414 w459] -> w22
      frame "假", Default {
      }
      frame "Good_Clear_NVM_Error" {
        n9 = Unbundle By Name(w60) -> ("Table"=w66:string[][], "daemon reference"=w71:refnum<k5>)
        n10 = call "Select_Table_Vaule Enable_Disable.vi"("Action"=w67, "Table"=w66) -> ("Enable"=w68:bool)  [unwired: 8 in, 1 out]
        n11 = case shown="假" w68 {
          tunnel: w71 -> [w78 w93]
          tunnel: [TRUE w83] -> _
          tunnel: [w78 w87] -> w57
          tunnel: [w77 w81] -> w62
          tunnel: w67 -> [_ w86]
          tunnel: w66 -> [_ w85]
          tunnel: [_ w82] -> w58
          tunnel: [w77 w81] -> w56
          tunnel: [w77 w80] -> w55
          frame False {
            w77 = "Skip" ("response")
          }
          frame True {
            w92 = "UIdisplay" ("Process (\"\" - local)")
            n12 = call "clear_nvm_error.vi"("daemon reference in"=w93) -> ("error out"=w82:errorcluster, "response"=w81:string, "daemon reference out"=w87:refnum<k5>)  [unwired: 7 in, 1 out]
            n13 = call "Select_Table_Vaule.vi"("Vaule"=w81, "Action"=w86, "Table"=w85) -> ("Result"=w83:bool, "vaule"=w84:string[])  [unwired: 7 in]
            n14 = Append True/False String(1:w83, 2:"FAIL" ("真字符串"), 3:"PASS" ("真字符串")) -> (0:w80:string)  [unwired: 1 in]
            n15 = Build Array (concatenate)(w84, w81, w80) -> (w91:string[])
            n16 = Flatten To XML(anything=w91) -> (xml string=w90:string)
            n17 = call "AMC Send Local Message.vi"("Process (\"\" - local)"=w92, "Message Value"=w90, "Message Name"=w92) -> ()  [unwired: 7 in, 2 out]
          }
        }
        n18 = call <vilib>:"Space Constant.vi"() -> ("String"=w70:string)
        n19 = Concatenate Strings(w67, w70, w62) -> (w69:string)
        n20 = Bundle By Name(cluster=w60, "daemon reference"=w57, "GOOD.GOOD UNIT - Clear EEPROM Error Log"=w56, "GOOD_Status.GOOD UNIT - Clear EEPROM Error Log"=w55) -> (w59:T1)
        n21 = call "LogStatus.vi"("error in (no error)"=w58, "last message"=w72, "message"=w69) -> ("error  out"=w73:errorcluster)  [unwired: 8 in]
        n22 = case shown="错误" w58 {
          tunnel: [_ TRUE] -> w63
          tunnel: [_ "Error"] -> w64
          frame No Error {
          }
          frame Error {
          }
        }
      }
      frame "Good_Write_Product_Timestamp(A)" {
        (unwired) timestamp(0 s since 1904-01-01)
        w109 = i64 0 ("default (0 I32)")
        n23 = Unbundle By Name(w120) -> ("Rig ID"=w119:string, "Tester ID"=w118:string, "PassMark Revision"=w117:string)
        n24 = Unbundle By Name(w104) -> ("Table"=w122:string[][], "daemon reference"=w129:refnum<k5>)
        n25 = Get Date/Time In Seconds() -> (seconds since 1Jan1904=w108:timestamp)
        n26 = Subtract(x=w108, y=timestamp(2082844800 s since 1904-01-01) ("x")) -> (x-y=w107:dbl)
        n27 = To Quad Integer(1:w107) -> (0:w105:i64)
        n28 = Decimal String To Number(string=w119, default (0L)=w109) -> (number=w116:i64)  [unwired: 1 in, 1 out]
        n29 = Decimal String To Number(string=w118, default (0L)=w109) -> (number=w115:i64)  [unwired: 1 in, 1 out]
        n30 = Decimal String To Number(string=w117, default (0L)=w109) -> (number=w114:i64)  [unwired: 1 in, 1 out]
        n31 = call "Select_Table_Vaule Enable_Disable.vi"("Action"=w123, "Table"=w122) -> ("Enable"=w124:bool)  [unwired: 8 in, 1 out]
        n32 = case shown="假" w124 {
          tunnel: w129 -> [w137 w155]
          tunnel: [TRUE w150] -> _
          tunnel: [w137 w154] -> w101
          tunnel: [w136 w142] -> w110
          tunnel: w123 -> [_ w153]
          tunnel: w122 -> [_ w152]
          tunnel: w116 -> [_ w147]
          tunnel: w115 -> [_ w146]
          tunnel: w114 -> [_ w145]
          tunnel: w105 -> [_ w143]
          tunnel: [_ w140] -> w113
          tunnel: [_ w144] -> w103
          tunnel: [_ w142] -> _
          tunnel: [w136 w141] -> w94
          tunnel: [T7 {"TIMESTAMP"="Skip", "RIG_ID"="Skip", "PASSMARK_ID"="Skip", "PASSMARK_REV"="Skip"} w139] -> w102
          frame False {
            w136 = "Skip" ("software string")
          }
          frame True {
            w160 = "UIdisplay" ("Process (\"\" - local)")
            n33 = Bundle By Name(cluster=T8 {"TIMESTAMP"=0, "RIG_ID"=0, "PASSMARK_ID"=0, "PASSMARK_REV"=0} ("Parameter"), "TIMESTAMP"=w143, "RIG_ID"=w147, "PASSMARK_ID"=w146, "PASSMARK_REV"=w145) -> (w140:T8)
            n34 = call "set_cal_info.vi"("Parameter"=w140, "Mode"=device_mode."PROD", "daemon reference in"=w155) -> ("error out"=w144:errorcluster, "response"=w142:string, "daemon reference out"=w154:refnum<k5>)  [unwired: 5 in, 1 out]
            n35 = call "Select_Table_Vaule.vi"("Vaule"=w142, "Action"=w153, "Table"=w152) -> ("Result"=w150:bool, "vaule"=w151:string[])  [unwired: 7 in]
            n36 = call "时间延迟"("error in (no error)"=w144) -> ()  [unwired: 10 in, 1 out]
            n37 = Append True/False String(1:w150, 2:"FAIL" ("真字符串"), 3:"PASS" ("真字符串")) -> (0:w141:string)  [unwired: 1 in]
            n38 = Build Array (concatenate)(w151, w142, w141) -> (w159:string[])
            n39 = Flatten To XML(anything=w159) -> (xml string=w158:string)
            n40 = Number To Decimal String(number=w140) -> (decimal integer string=w139:T7)  [unwired: 1 in]
            n41 = call "AMC Send Local Message.vi"("Process (\"\" - local)"=w160, "Message Value"=w158, "Message Name"=w160) -> ()  [unwired: 7 in, 2 out]
          }
        }
        n42 = call <vilib>:"Space Constant.vi"() -> ("String"=w126:string)
        n43 = Concatenate Strings(w123, w126, w110) -> (w125:string)
        n44 = Unbundle By Name(w102) -> ("TIMESTAMP"=w98:string, "RIG_ID"=w97:string, "PASSMARK_ID"=w96:string, "PASSMARK_REV"=w95:string)
        n45 = Bundle By Name(cluster=w104, "daemon reference"=w101, "GOOD.GOOD UNIT - Write Product Timestamp - Mode"="PROD", "GOOD.GOOD UNIT - Write Product Timestamp - Timestamp"=w98, "GOOD.GOOD UNIT - Write Product Timestamp - Rig ID"=w97, "GOOD.GOOD UNIT - Write Product Timestamp - Passmark ID"=w96, "GOOD.GOOD UNIT - Write Product Timestamp - Passmark Rev"=w95, "GOOD_Status.GOOD UNIT - Write Product Timestamp - Mode"=w94, "GOOD_Status.GOOD UNIT - Write Product Timestamp - Timestamp"=w94, "GOOD_Status.GOOD UNIT - Write Product Timestamp - Rig ID"=w94, "GOOD_Status.GOOD UNIT - Write Product Timestamp - Passmark ID"=w94, "GOOD_Status.GOOD UNIT - Write Product Timestamp - Passmark Rev"=w94) -> (w100:T1)
        n46 = Bundle By Name(cluster=w128, "good.Write_Product_TS"=w113) -> (w127:T3)
        n47 = call "LogStatus.vi"("error in (no error)"=w103, "last message"=w130, "message"=w125) -> ("error  out"=w131:errorcluster)  [unwired: 8 in]
        n48 = case shown="错误" w103 {
          tunnel: [_ TRUE] -> w111
          tunnel: [_ "Error"] -> w112
          frame No Error {
          }
          frame Error {
          }
        }
      }
      frame "Good_Set_DDM_to_Product_mode" {
        n49 = Unbundle By Name(w166) -> ("Table"=w172:string[][], "daemon reference"=w177:refnum<k5>)
        n50 = call "Select_Table_Vaule Enable_Disable.vi"("Action"=w173, "Table"=w172) -> ("Enable"=w171:bool)  [unwired: 8 in, 1 out]
        n51 = case shown="假" w171 {
          tunnel: w177 -> [w184 w195]
          tunnel: [w184 w194] -> w163
          tunnel: [w183 w187] -> w168
          tunnel: w173 -> [_ w193]
          tunnel: w172 -> [_ w192]
          tunnel: [_ w188] -> w165
          tunnel: [_ w187] -> _
          tunnel: [w183 w186] -> w162
          tunnel: [w183 "PROD"] -> w161
          frame False {
            w183 = "Skip" ("software string")
            (unwired) TRUE
          }
          frame True {
            w200 = "UIdisplay" ("Process (\"\" - local)")
            n52 = call "set_device_mode.vi"("Mode"=device_mode."PROD", "daemon reference in"=w195) -> ("error out"=w188:errorcluster, "response"=w187:string, "daemon reference out"=w194:refnum<k5>)  [unwired: 6 in, 1 out]
            n53 = call "Select_Table_Vaule.vi"("Vaule"=w187, "Action"=w193, "Table"=w192) -> ("Result"=w190:bool, "vaule"=w191:string[])  [unwired: 7 in]
            n54 = call "时间延迟2"("error in (no error)"=w188) -> ()  [unwired: 10 in, 1 out]
            n55 = Append True/False String(1:w190, 2:"FAIL" ("真字符串"), 3:"PASS" ("真字符串")) -> (0:w186:string)  [unwired: 1 in]
            n56 = Build Array (concatenate)(w191, w187, w186) -> (w199:string[])
            n57 = Flatten To XML(anything=w199) -> (xml string=w198:string)
            n58 = call "AMC Send Local Message.vi"("Process (\"\" - local)"=w200, "Message Value"=w198, "Message Name"=w200) -> ()  [unwired: 7 in, 2 out]
          }
        }
        n59 = call <vilib>:"Space Constant.vi"() -> ("String"=w176:string)
        n60 = Concatenate Strings(w173, w176, w168) -> (w175:string)
        n61 = Bundle By Name(cluster=w166, "GOOD_Status.GOOD UNIT - Set Device Mode to PROD"=w162, "GOOD.GOOD UNIT - Set Device Mode to PROD"=w161, "daemon reference"=w163) -> (w164:T1)
        n62 = call "LogStatus.vi"("error in (no error)"=w165, "last message"=w178, "message"=w175) -> ("error  out"=w179:errorcluster)  [unwired: 8 in]
        n63 = case shown="错误" w165 {
          tunnel: [_ TRUE] -> w169
          tunnel: [_ "Error"] -> w170
          frame No Error {
          }
          frame Error {
          }
        }
      }
      frame "Good_Read_Product_Timestamp" {
        n64 = Unbundle By Name(w206) -> ("Table"=w208:string[][], "daemon reference"=w207:refnum<k5>)
        n65 = Unbundle By Name(w219) -> ("good.Write_Product_TS.TIMESTAMP"=w211:i64)
        n66 = call "Select_Table_Vaule Enable_Disable.vi"("Action"=w215, "Table"=w208) -> ("Enable"=w214:bool)  [unwired: 8 in, 1 out]
        n67 = case shown="真" w214 {
          tunnel: w207 -> [w230 w248]
          tunnel: [w230 w247] -> w202
          tunnel: ["" ("software string") w232] -> w209
          tunnel: w215 -> [_ w246]
          tunnel: w208 -> [_ w245]
          tunnel: [_ w234] -> w204
          tunnel: [_ w237] -> w205
          tunnel: w211 -> [_ w235]
          tunnel: [_ w233] -> w203
          tunnel: [_ w232] -> _
          tunnel: [_ w231] -> _
          frame False {
            (unwired) TRUE
          }
          frame True {
            w253 = "UIdisplay" ("Process (\"\" - local)")
            n68 = call "get_cal_info.vi"("Mode"=device_mode."PROD", "daemon reference in"=w248) -> ("error out"=w237:errorcluster, "response"=w232:string, "daemon reference out"=w247:refnum<k5>)  [unwired: 5 in, 2 out]
            n69 = call "Select_Table_Vaule.vi"("Vaule"=w232, "Action"=w246, "Table"=w245) -> ("Result"=w243:bool, "vaule"=w244:string[])  [unwired: 7 in]
            n70 = Spreadsheet String To Array(delimiter (Tab)="," ("分隔符(Tab)"), format string="" ("格式字符串"), spreadsheet string=w232, array type (2D Dbl)=i64[] []) -> (array=w239:i64[])
            n71 = Array To Cluster(array=w239) -> (cluster=w234:T13)
            n72 = Append True/False String(1:w243, 2:"FAIL" ("真字符串"), 3:"PASS" ("真字符串")) -> (0:w231:string)  [unwired: 1 in]
            n73 = Build Array (concatenate)(w244, w232, w231) -> (w252:string[])
            n74 = Flatten To XML(anything=w252) -> (xml string=w251:string)
            n75 = Unbundle By Name(w234) -> ("[0]"=w236:i64)
            n76 = call "AMC Send Local Message.vi"("Process (\"\" - local)"=w253, "Message Value"=w251, "Message Name"=w253) -> ()  [unwired: 7 in, 2 out]
            n77 = Equal?(x=w236, y=w235) -> (x = y?=w233:bool)
          }
        }
        n78 = call <vilib>:"Space Constant.vi"() -> ("String"=w217:string)
        n79 = Concatenate Strings(w215, w217, w209) -> (w216:string)
        n80 = case shown="错误" w205 {
          tunnel: [w224 "Error"] -> w213
          tunnel: w203 -> [w223 _]
          tunnel: [w223 FALSE] -> w210
          frame No Error {
            n81 = Select(t="Good_Backup_DDM_NVM", s=w223, f="Finalization_NG_unit") -> (s? t:f=w224:string)
          }
          frame Error {
          }
        }
        n82 = Bundle By Name(cluster=w206, "daemon reference"=w202) -> (w201:T1)
        n83 = Bundle By Name(cluster=w219, "good.Read_Product_TS"=w204) -> (w218:T3)
        n84 = call "LogStatus.vi"("error in (no error)"=w205, "last message"=w220, "message"=w216) -> ("error  out"=w221:errorcluster)  [unwired: 8 in]
        n85 = Not(x=w210) -> (.not. x?=w212:bool)
      }
      frame "Good_Backup_DDM_NVM" {
        w272 = "_" ("string")
        n86 = Unbundle By Name(w259) -> ("Table"=w283:string[][], "daemon reference"=w287:refnum<k5>, "Config"=w281:string[][], "SN"=w269:string)
        n87 = call "PathChoose.vi"(11:PathChoose."backup_nvm") -> ("Path_Out"=w271:path)  [unwired: 10 in]
        n88 = Path To String(path=w271) -> (string=w270:string)
        n89 = Format Date/Time String(time format string (%c)="%Y%m%d%H%M%S" ("时间格式字符串(%c)")) -> (date/time string=w268:string)  [unwired: 2 in]
        n90 = call "Select_Table_Vaule Enable_Disable.vi"("Action"=w284, "Table"=w283) -> ("Enable"=w282:bool)  [unwired: 8 in, 1 out]
        n91 = Concatenate Strings(w270, "\\" ("字符串"), w269, w272, w268, w272, "CAL" ("时间格式字符串(%c)"), ".json" ("string")) -> (w275:string)
        n92 = String To Path(string=w275) -> (path=w263:path)
        n93 = call <vilib>:"Check if File or Folder Exists.vi"("path"=w263) -> ("error out"=w265:errorcluster, "file or folder exists?"=w264:bool, "dup path"=w266:path)  [unwired: 8 in]
        n94 = case shown="假" w264 {
          tunnel: w265 -> [w294 w295]
          tunnel: w266 -> [w291 w296]
          tunnel: [w291 w296] -> w262
          tunnel: [w293 w295] -> _
          frame False {
            n95 = Open/Create/Replace File(file path (use dialog)=w291, error in=w294, operation (0:open)=T11."create") -> (error out=w293:errorcluster)  [unwired: 3 in, 2 out]
          }
          frame True {
          }
        }
        n96 = case shown="假" w282 {
          tunnel: w287 -> [w300 w311]
          tunnel: [w300 w310] -> w257
          tunnel: [w299 w302] -> w261
          tunnel: w284 -> [_ w309]
          tunnel: w283 -> [_ w308]
          tunnel: w281 -> [_ _]
          tunnel: [_ w306] -> _
          tunnel: [_ w304] -> w258
          tunnel: w262 -> [_ w303]
          tunnel: [w299 w302] -> w255
          tunnel: [w299 w301] -> w254
          frame False {
            w299 = "Skip" ("software string")
            (unwired) TRUE
          }
          frame True {
            w316 = "UIdisplay" ("Process (\"\" - local)")
            n97 = call "backup_nvm.vi"("type"=read_nvm_section."CAL", "File Path"=w303, "daemon reference in"=w311) -> ("error out"=w304:errorcluster, "response"=w302:string, "daemon reference out"=w310:refnum<k5>)  [unwired: 5 in, 1 out]
            n98 = call "Select_Table_Vaule.vi"("Vaule"=w302, "Action"=w309, "Table"=w308) -> ("Result"=w306:bool, "vaule"=w307:string[])  [unwired: 7 in]
            n99 = Append True/False String(1:w306, 2:"FAIL" ("真字符串"), 3:"PASS" ("真字符串")) -> (0:w301:string)  [unwired: 1 in]
            n100 = Build Array (concatenate)(w307, w302, w301) -> (w315:string[])
            n101 = Flatten To XML(anything=w315) -> (xml string=w314:string)
            n102 = call "AMC Send Local Message.vi"("Process (\"\" - local)"=w316, "Message Value"=w314, "Message Name"=w316) -> ()  [unwired: 7 in, 2 out]
          }
        }
        n103 = call <vilib>:"Space Constant.vi"() -> ("String"=w286:string)
        n104 = Concatenate Strings(w284, w286, w261) -> (w285:string)
        n105 = Bundle By Name(cluster=w259, "daemon reference"=w257, "GOOD.GOOD UNIT - Backup PCBA Calibration EEPROM Response"=w255, "GOOD_Status.GOOD UNIT - Backup PCBA Calibration EEPROM Response"=w254) -> (w256:T1)
        n106 = call "LogStatus.vi"("error in (no error)"=w258, "last message"=w288, "message"=w285) -> ("error  out"=w289:errorcluster)  [unwired: 8 in]
        n107 = case shown="错误" w258 {
          tunnel: [_ TRUE] -> w277
          tunnel: [_ "Error"] -> w278
          frame No Error {
          }
          frame Error {
          }
        }
      }
      frame "Good_Check_Secuity_Bit" {
        (unwired) "Good_Set_Secuity_Bit"
        n108 = Unbundle By Name(w322) -> ("Table"=w329:string[][], "daemon reference"=w335:refnum<k5>, "Config"=w328:string[][])
        n109 = call "Select_Table_Vaule Enable_Disable.vi"("Action"=w330, "Table"=w329) -> ("Enable"=w325:bool)  [unwired: 8 in, 1 out]
        n110 = case shown="假" w325 {
          tunnel: w335 -> [w348 w354]
          tunnel: [w348 w353] -> w320
          tunnel: [w346 w350] -> w326
          tunnel: w330 -> [_ w357]
          tunnel: w329 -> [_ w356]
          tunnel: w328 -> [_ _]
          tunnel: [TRUE w352] -> w324
          tunnel: [_ w351] -> w321
          tunnel: [w346 w350] -> w318
          tunnel: [w346 w349] -> w317
          frame False {
            w346 = "Skip" ("software string")
          }
          frame True {
            w362 = "UIdisplay" ("Process (\"\" - local)")
            n111 = call "get_security_bit.vi"("daemon reference in"=w354) -> ("error out"=w351:errorcluster, "response"=w350:string, "daemon reference out"=w353:refnum<k5>)  [unwired: 7 in, 1 out]
            n112 = call "Select_Table_Vaule.vi"("Vaule"=w350, "Action"=w357, "Table"=w356) -> ("Result"=w352:bool, "vaule"=w355:string[])  [unwired: 7 in]
            n113 = Append True/False String(1:w352, 2:"FAIL" ("真字符串"), 3:"PASS" ("真字符串")) -> (0:w349:string)  [unwired: 1 in]
            n114 = Build Array (concatenate)(w355, w350, w349) -> (w361:string[])
            n115 = Flatten To XML(anything=w361) -> (xml string=w360:string)
            n116 = call "AMC Send Local Message.vi"("Process (\"\" - local)"=w362, "Message Value"=w360, "Message Name"=w362) -> ()  [unwired: 7 in, 2 out]
          }
        }
        n117 = call <vilib>:"Space Constant.vi"() -> ("String"=w332:string)
        n118 = Concatenate Strings(w330, w332, w326) -> (w331:string)
        n119 = Bundle By Name(cluster=w322, "daemon reference"=w320, "GOOD.GOOD UNIT - Check Security Bit"=w318, "GOOD_Status.GOOD UNIT - Check Security Bit"=w317) -> (w319:T1)
        n120 = case shown="无错误" w321 {
          tunnel: [w339 TRUE] -> w327
          tunnel: [w341 "Error"] -> w323
          tunnel: w324 -> [w340 _]
          frame No Error {
            n121 = Select(t="Good_Set_Calibration_Lock", s=w340, f="Finalization_NG_unit") -> (s? t:f=w341:string)
            n122 = Not(x=w340) -> (.not. x?=w339:bool)
          }
          frame Error {
          }
        }
        n123 = Bundle By Name(cluster=w334, "good.Good_Check_Secuity_Bit_Stauts"=w324) -> (w333:T3)
        n124 = call "LogStatus.vi"("error in (no error)"=w321, "last message"=w336, "message"=w331) -> ("error  out"=w337:errorcluster)  [unwired: 8 in]
      }
      frame "Good_Set_Secuity_Bit" {
        n125 = Unbundle By Name(w367) -> ("Table"=w374:string[][], "daemon reference"=w378:refnum<k5>, "Config"=w373:string[][])
        n126 = call "Select_Table_Vaule Enable_Disable.vi"("Action"=w375, "Table"=w374) -> ()  [unwired: 8 in, 2 out]
        n127 = case shown="假" FALSE {
          tunnel: w378 -> [w395 w401]
          tunnel: [w395 w400] -> w365
          tunnel: [w384 w397] -> w369
          tunnel: w375 -> [w386 w404]
          tunnel: w374 -> [w387 w403]
          tunnel: w373 -> [_ _]
          tunnel: [w385 w399] -> _
          tunnel: [_ w398] -> w366
          tunnel: [_ w397] -> _
          tunnel: [_ w396] -> _
          frame False {
            w394 = "UIdisplay" ("Process (\"\" - local)")
            w384 = "Disable" ("software string")
            w385 = TRUE
            n128 = call "Select_Table_Vaule.vi"("Action"=w386, "Table"=w387) -> ("vaule"=w388:string[])  [unwired: 8 in, 1 out]
            n129 = Append True/False String(1:w385, 2:"FAIL" ("真字符串"), 3:"PASS" ("真字符串")) -> (0:w389:string)  [unwired: 1 in]
            n130 = Build Array (concatenate)(w388, w384, w389) -> (w393:string[])
            n131 = Flatten To XML(anything=w393) -> (xml string=w392:string)
            n132 = call "AMC Send Local Message.vi"("Process (\"\" - local)"=w394, "Message Value"=w392, "Message Name"=w394) -> ()  [unwired: 7 in, 2 out]
          }
          frame True {
            w409 = "UIdisplay" ("Process (\"\" - local)")
            n133 = call "set_security_bit.vi"("daemon reference in"=w401) -> ("error out"=w398:errorcluster, "response"=w397:string, "daemon reference out"=w400:refnum<k5>)  [unwired: 7 in, 1 out]
            n134 = call "Select_Table_Vaule.vi"("Vaule"=w397, "Action"=w404, "Table"=w403) -> ("Result"=w399:bool, "vaule"=w402:string[])  [unwired: 7 in]
            n135 = Append True/False String(1:w399, 2:"FAIL" ("真字符串"), 3:"PASS" ("真字符串")) -> (0:w396:string)  [unwired: 1 in]
            n136 = Build Array (concatenate)(w402, w397, w396) -> (w408:string[])
            n137 = Flatten To XML(anything=w408) -> (xml string=w407:string)
            n138 = call "AMC Send Local Message.vi"("Process (\"\" - local)"=w409, "Message Value"=w407, "Message Name"=w409) -> ()  [unwired: 7 in, 2 out]
          }
        }
        n139 = call <vilib>:"Space Constant.vi"() -> ("String"=w377:string)
        n140 = Concatenate Strings(w375, w377, w369) -> (w376:string)
        n141 = Bundle By Name(cluster=w367, "daemon reference"=w365) -> (w364:T1)
        n142 = call "LogStatus.vi"("error in (no error)"=w366, "last message"=w379, "message"=w376) -> ("error  out"=w380:errorcluster)  [unwired: 8 in]
        n143 = case shown="错误" w366 {
          tunnel: [_ TRUE] -> w370
          tunnel: [_ "Error"] -> w371
          frame No Error {
          }
          frame Error {
          }
        }
      }
      frame "Good_Set_Calibration_Lock" {
        n144 = Unbundle By Name(w415) -> ("Table"=w421:string[][], "daemon reference"=w425:refnum<k5>, "Config"=w420:string[][])
        n145 = call "Select_Table_Vaule Enable_Disable.vi"("Action"=w422, "Table"=w421) -> ("Enable"=w417:bool)  [unwired: 8 in, 1 out]
        n146 = case shown="真" w417 {
          tunnel: w425 -> [w438 w444]
          tunnel: [w438 w443] -> w413
          tunnel: [w431 w441] -> w418
          tunnel: w422 -> [w432 w448]
          tunnel: w421 -> [w433 w447]
          tunnel: w420 -> [_ _]
          tunnel: [_ w439] -> w416
          tunnel: [w431 w441] -> w411
          tunnel: [w431 w440] -> w410
          frame False {
            w437 = "UIdisplay" ("Process (\"\" - local)")
            w431 = "Skip" ("software string")
            n147 = call "Select_Table_Vaule.vi"("Vaule"=w431, "Action"=w432, "Table"=w433) -> ("vaule"=w434:string[])  [unwired: 7 in, 1 out]
            n148 = Build Array (concatenate)(w434, w431, w431) -> (w436:string[])
            n149 = Flatten To XML(anything=w436) -> (xml string=w435:string)
            n150 = call "AMC Send Local Message.vi"("Process (\"\" - local)"=w437, "Message Value"=w435, "Message Name"=w437) -> ()  [unwired: 7 in, 2 out]
          }
          frame True {
            w453 = "UIdisplay" ("Process (\"\" - local)")
            n151 = call "set_calibration_lock.vi"("daemon reference in"=w444) -> ("error out"=w442:errorcluster, "response"=w441:string, "daemon reference out"=w443:refnum<k5>)  [unwired: 7 in, 1 out]
            n152 = call "时间延迟3"("error in (no error)"=w442) -> ("error out"=w439:errorcluster)  [unwired: 10 in]
            n153 = call "Select_Table_Vaule.vi"("Vaule"=w441, "Action"=w448, "Table"=w447) -> ("Result"=w445:bool, "vaule"=w446:string[])  [unwired: 7 in]
            n154 = Append True/False String(1:w445, 2:"FAIL" ("真字符串"), 3:"PASS" ("真字符串")) -> (0:w440:string)  [unwired: 1 in]
            n155 = Build Array (concatenate)(w446, w441, w440) -> (w452:string[])
            n156 = Flatten To XML(anything=w452) -> (xml string=w451:string)
            n157 = call "AMC Send Local Message.vi"("Process (\"\" - local)"=w453, "Message Value"=w451, "Message Name"=w453) -> ()  [unwired: 7 in, 2 out]
          }
        }
        n158 = call <vilib>:"Space Constant.vi"() -> ("String"=w424:string)
        n159 = Concatenate Strings(w422, w424, w418) -> (w423:string)
        n160 = case shown="无错误" w416 {
          tunnel: ["GOOD_UNIT_Get_Calibration_Lock" "Error"] -> w419
          frame No Error {
          }
          frame Error {
          }
        }
        n161 = Bundle By Name(cluster=w415, "daemon reference"=w413, "GOOD.GOOD UNIT - Set Calibration Lock"=w411, "GOOD_Status.GOOD UNIT - Set Calibration Lock"=w410) -> (w414:T1)
        n162 = call "LogStatus.vi"("error in (no error)"=w416, "last message"=w426, "message"=w423) -> ("error  out"=w427:errorcluster)  [unwired: 8 in]
      }
      frame "GOOD_UNIT_Get_Calibration_Lock" {
        (unwired) "Good_Set_Secuity_Bit"
        n163 = Unbundle By Name(w462) -> ("Table"=w467:string[][], "daemon reference"=w471:refnum<k5>, "Config"=w466:string[][])
        n164 = call "Select_Table_Vaule Enable_Disable.vi"("Action"=w468, "Table"=w467) -> ("Enable"=w464:bool)  [unwired: 8 in, 1 out]
        n165 = case shown="真" w464 {
          tunnel: w471 -> [w488 w494]
          tunnel: [w488 w493] -> w460
          tunnel: [w480 w490] -> w465
          tunnel: w468 -> [w481 w497]
          tunnel: w467 -> [w482 w496]
          tunnel: w466 -> [_ _]
          tunnel: [TRUE w492] -> w454
          tunnel: [_ w491] -> w461
          tunnel: [w480 w490] -> w458
          tunnel: [w480 w489] -> w457
          frame False {
            w486 = "UIdisplay" ("Process (\"\" - local)")
            w480 = "Skip" ("software string")
            n166 = call "Select_Table_Vaule.vi"("Vaule"=w480, "Action"=w481, "Table"=w482) -> ("vaule"=w483:string[])  [unwired: 7 in, 1 out]
            n167 = Build Array (concatenate)(w483, w480, w480) -> (w485:string[])
            n168 = Flatten To XML(anything=w485) -> (xml string=w484:string)
            n169 = call "AMC Send Local Message.vi"("Process (\"\" - local)"=w486, "Message Value"=w484, "Message Name"=w486) -> ()  [unwired: 7 in, 2 out]
          }
          frame True {
            w502 = "UIdisplay" ("Process (\"\" - local)")
            n170 = call "get_calibration_lock.vi"("daemon reference in"=w494) -> ("error out"=w491:errorcluster, "response"=w490:string, "daemon reference out"=w493:refnum<k5>)  [unwired: 7 in, 1 out]
            n171 = call "Select_Table_Vaule.vi"("Vaule"=w490, "Action"=w497, "Table"=w496) -> ("Result"=w492:bool, "vaule"=w495:string[])  [unwired: 7 in]
            n172 = Append True/False String(1:w492, 2:"FAIL" ("真字符串"), 3:"PASS" ("真字符串")) -> (0:w489:string)  [unwired: 1 in]
            n173 = Build Array (concatenate)(w495, w490, w489) -> (w501:string[])
            n174 = Flatten To XML(anything=w501) -> (xml string=w500:string)
            n175 = call "AMC Send Local Message.vi"("Process (\"\" - local)"=w502, "Message Value"=w500, "Message Name"=w502) -> ()  [unwired: 7 in, 2 out]
          }
        }
        n176 = call <vilib>:"Space Constant.vi"() -> ("String"=w470:string)
        n177 = Concatenate Strings(w468, w470, w465) -> (w469:string)
        n178 = Bundle By Name(cluster=w462, "daemon reference"=w460, "GOOD.GOOD UNIT - Get_Calibration_Lock"=w458, "GOOD_Status.GOOD UNIT - Get_Calibration_Lock"=w457, "OK/NG"=w454) -> (w459:T1)
        n179 = case shown="无错误" w461 {
          tunnel: [w477 "Error"] -> w463
          tunnel: w454 -> [w476 _]
          frame No Error {
            n180 = Select(t="Disconnect_UUT", s=w476, f="Finalization_NG_unit") -> (s? t:f=w477:string)
          }
          frame Error {
          }
        }
        n181 = call "LogStatus.vi"("error in (no error)"=w461, "last message"=w472, "message"=w469) -> ("error  out"=w473:errorcluster)  [unwired: 8 in]
      }
    }
    n182 = call "6-AlarmStatus.vi"("Step"=enum16{"Initial", "Write", "Read"}."Read") -> ("AlarmValue Out"=w20:bool[])  [unwired: 9 in, 1 out]
    n183 = call "Stop.vi"("Step"=enum16{"Initial", "Write", "Read"}."Read") -> ("Stop Out"=w28:bool)  [unwired: 9 in, 1 out]
    n184 = call "Exit.vi"("Step"=enum16{"Initial", "Write", "Read"}."Read" ("step")) -> ("Exit Out"=w27:bool)  [unwired: 9 in, 1 out]
    n185 = Or Array Elements(Boolean array=w20) -> (logical OR=w19:bool)
    n186 = Compound Arithmetic op=OR(w26, w28, w27, w19) -> (w25:bool)
    n187 = call "AMC Run Step.vi"("Message Queue In"=w47, "Message Name"=w35, "Message Value"=w33, "error in (no error)"=w42, "Mli/Sig"=FALSE) -> ("Message Queue Out"=w46:T4, "error out"=w41:errorcluster)  [unwired: 13 in]
  }
  "Message Queue Out" <- w6
  "error out" <- w5
  "Data" <- w12
  "Flow" <- w9
  "Data out" <- w1
